vi "PLC版CODMn数据插入.vi"(0 "data":T2={"时间"=timestamp(0 s since 1904-01-01), "测量模式"="水样测试", "数据类型"="N", "检测值"=0.0, "单位"="mg/L", "数据标识"="N", "高锰酸钾滴定数"=0.0, "量程"=0.0, "序列号"="", "标样参考值"=0.0, "跨度值"=0.0, "高锰酸钾原始滴定数"=0.0, "ORPA"=0.0, "ORPB"=0.0, "ORPK"=0.0, "COD滴定值"=0.0, "温度"=0.0, "因子编码"="", "测量量程"=0.0, "测量精度"=0.0, "测量间隔"=0.0, "消解温度"=0.0, "消解时长"=0.0, "空白校准时间"=timestamp(0 s since 1904-01-01), "曲线截距"=0.0, "曲线斜率"=0.0, "测量检出限"=0.0, "测量信号值"=0.0, "线性相关系数"=0.0, "二次多项式系数"=0.0, "标样校准时间"=timestamp(0 s since 1904-01-01), "稀释倍数"=0.0, "三项式系数"=0.0, "量程系数"=0.0, "LastTime"=timestamp(0 s since 1904-01-01)}, 1 "Password":string, 3 "错误输入（无错误）":errorcluster, 4 "数据库类型":T1) -> (10 "错误输出":errorcluster)   [LabVIEW 2016]
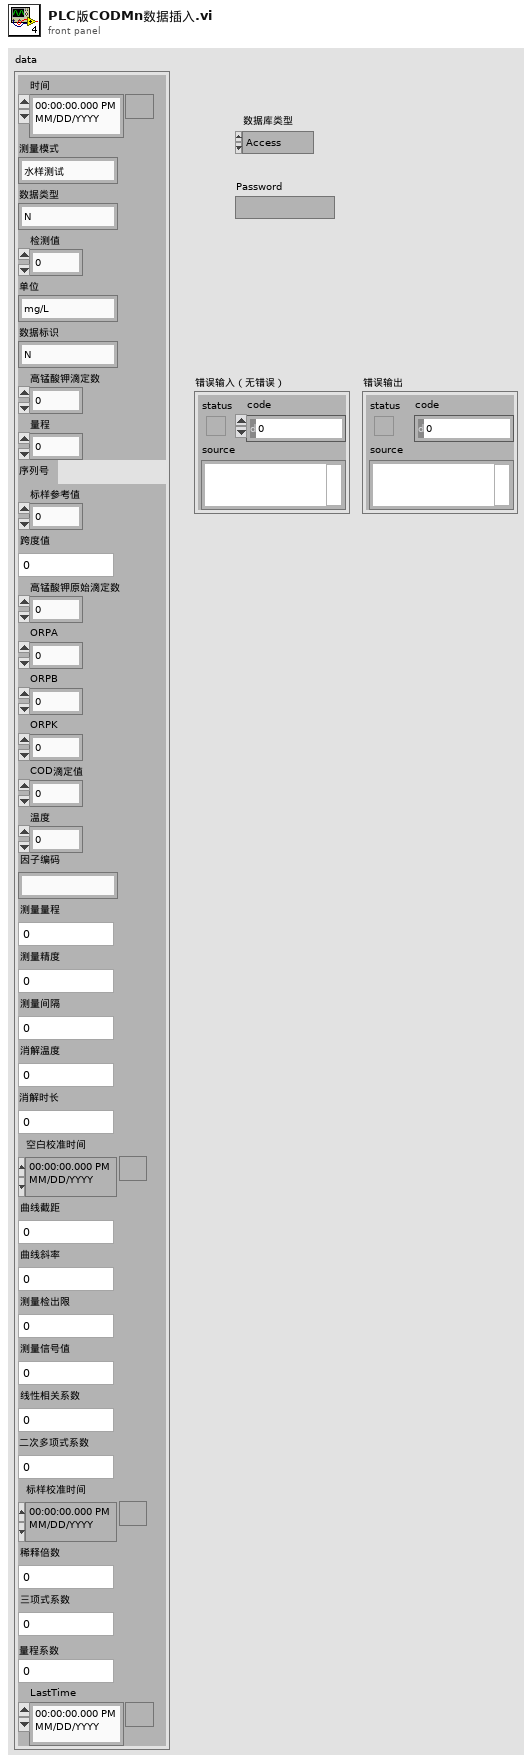
[diagram p1: front panel]
types:
  T1 = typedef "数据库类型.ctl" = enum16{"Access", "SQLite"}
  T2 = typedef "PLC版 CODMn字段定义.ctl" = cluster{"时间":timestamp, "测量模式":string, "数据类型":string, "检测值":sgl, "单位":string, "数据标识":string, "高锰酸钾滴定数":sgl, "量程":sgl, "序列号":string, "标样参考值":sgl, "跨度值":sgl, "高锰酸钾原始滴定数":sgl, "ORPA":sgl, "ORPB":sgl, "ORPK":sgl, "COD滴定值":sgl, "温度":sgl, "因子编码":string, "测量量程":sgl, "测量精度":sgl, "测量间隔":sgl, "消解温度":sgl, "消解时长":sgl, "空白校准时间":timestamp, "曲线截距":sgl, "曲线斜率":sgl, "测量检出限":sgl, "测量信号值":sgl, "线性相关系数":sgl, "二次多项式系数":sgl, "标样校准时间":timestamp, "稀释倍数":sgl, "三项式系数":sgl, "量程系数":sgl, "LastTime":timestamp}
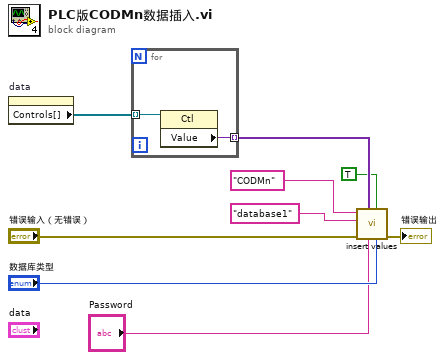
[diagram p0: block diagram]
diagram:
  n1 = property on="data" class="Clust (严格)"() -> ("Controls[]"=w9:refnum<vi>[])  [unwired: 2 in, 2 out]
  n2 = for {
    tunnel: w9 -> [w11] mode=indexing
    tunnel: [w10] -> w8 mode=indexing
    n3 = property class="Ctl"(reference=w11) -> ("Value"=w10:variant)  [unwired: 1 in, 2 out]
  }
  n4 = call "insert values.vi"("数据库类型"="数据库类型", "是否创建唯一键"=TRUE, "Password"="Password", "data"=w8, "错误输入（无错误）"="错误输入（无错误）", "database"="database1", "Tabe Name"="CODMn") -> ("错误输出"=→"错误输出":errorcluster)  [unwired: 4 in]
